vi "Login (Start Here!).vi"() -> ()   [LabVIEW 2012]
panel:
  out "error out":errorcluster
  in  "stop":bool
  out "Incorrect!":bool
  out "Verified!":bool
  in  "OK":bool
  in  "Password":string
  in  "User Name":string
  # "EXO Login"
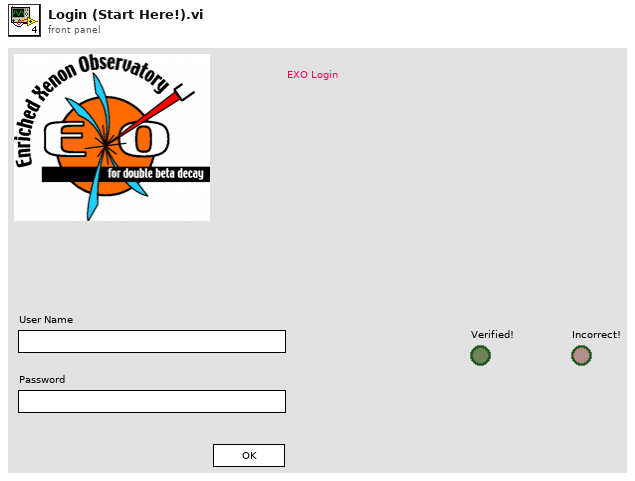
[diagram p1: front panel]
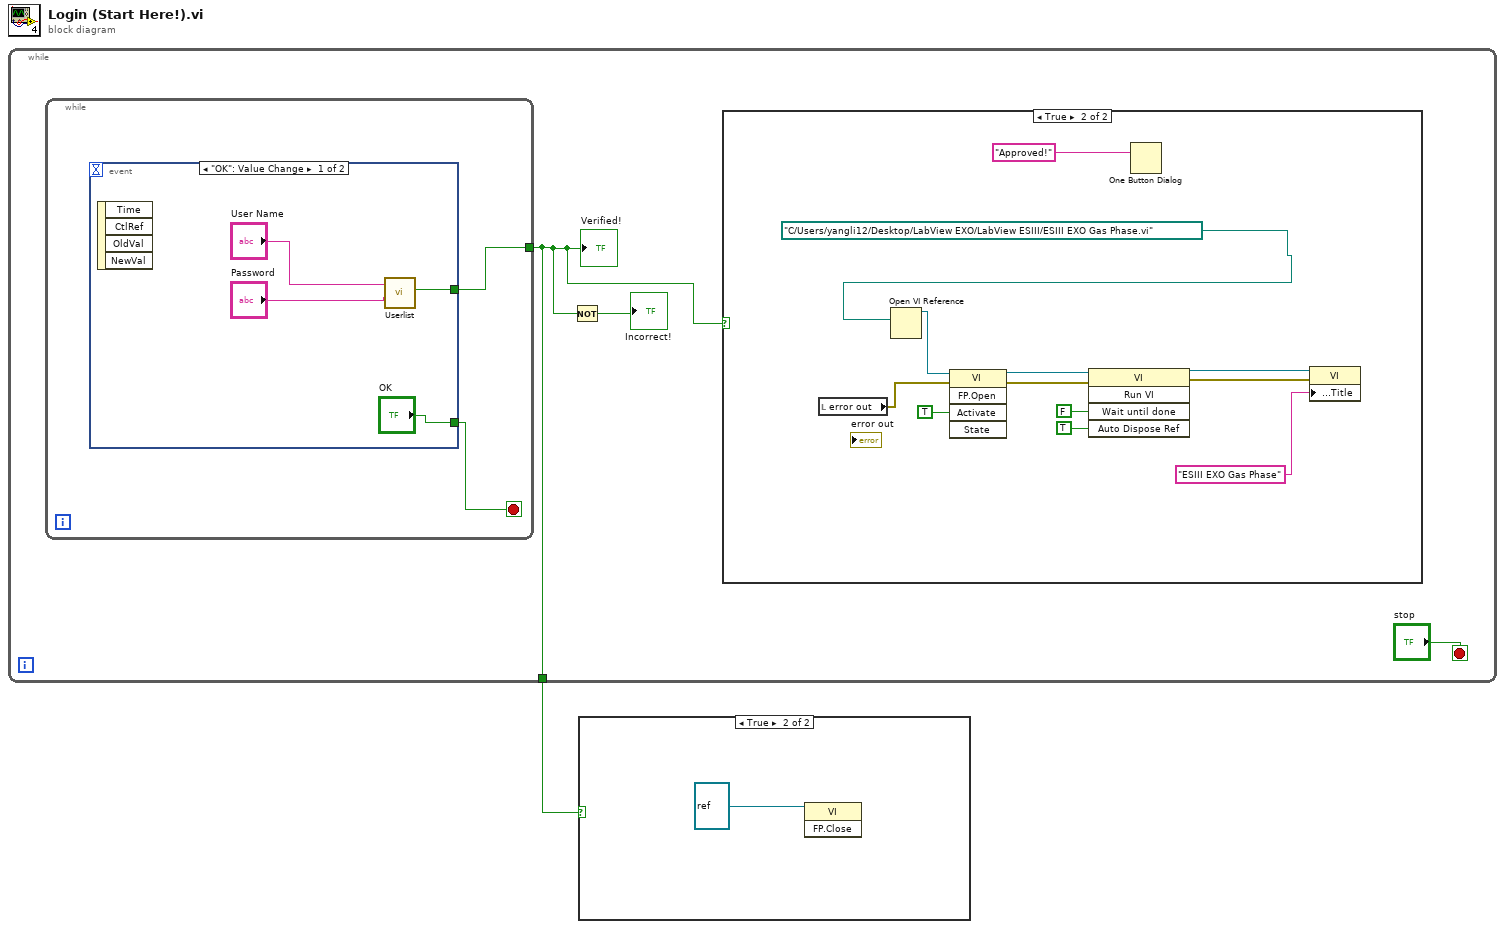
[diagram p0: block diagram]
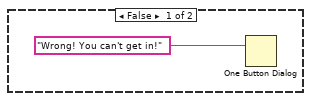
[diagram p3: hidden frame]
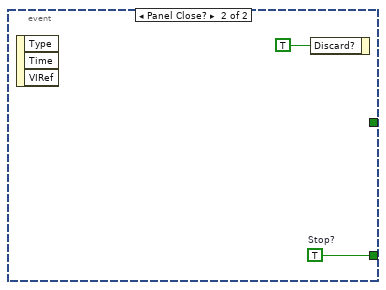
[diagram p4: hidden frame]
diagram:
  n1 = while {
    tunnel: [w2] -> w1
    stop <- "stop" stop-if-true
    n2 = while {
      tunnel: [w19] -> w2
      stop <- w18 stop-if-true
      n3 = event shown="[0] \"OK\": Value Change" {
        selector: _ -> [_ _]
        dyn-events: _ -> [_ _]
        timeout: _ -> [_ _]
        tunnel: ["OK" w24] -> w18
        tunnel: [w20 _] -> w19
        event "OK": Value Change {
          n4 = event-data() -> ()  [unwired: 1 in, 4 out]
          n5 = call "Userlist.vi"("Password"="Password", "Login"="User Name") -> ("Verified?"=w20:bool)  [unwired: 9 in]
        }
        event Panel Close? {
          w24 = TRUE  # Stop?
          n6 = event-data() -> ()  [unwired: 1 in, 3 out]
          n7 = event-data("Discard?"=TRUE) -> ()  [unwired: 1 in, 1 out]
        }
      }
    }
    "Verified!" <- w2
    n8 = Not(x=w2) -> (.not. x?=→"Incorrect!":bool)
    n9 = case shown="True" w2 {
      frame False {
        n10 = One Button Dialog(message="Wrong! You can't get in!" ("String 2")) -> ()  [unwired: 2 out]
      }
      frame True {
        n11 = local read "error out"() -> (w13:errorcluster)
        n12 = Open VI Reference(vi path=path "C:/Users/yangli12/Desktop/LabView EXO/LabView ESIII/ESIII EXO Gas Phase.vi") -> (vi reference=w16:refnum<vi>)  [unwired: 5 in, 1 out]
        n13 = invoke class="VI" method="FP.Open"(reference=w16, error in=w13, "Activate"=TRUE ("Activate?")) -> (reference out=w14:refnum<vi>, error out=w12:errorcluster)  [unwired: 2 in, 3 out]
        n14 = invoke class="VI" method="Run VI"(reference=w14, error in=w12, "Wait until done"=FALSE ("Wait Until Done"), "Auto Dispose Ref"=TRUE ("Auto Dispose Reference")) -> (reference out=w8:refnum<vi>, error out=w9:errorcluster)  [unwired: 1 in, 3 out]
        n15 = One Button Dialog(message="Approved!" ("String 2")) -> ()  [unwired: 2 out]
        n16 = property class="VI"(reference=w8, error in=w9, "Front Panel.Title"="ESIII EXO Gas Phase" ("Front Panel Window:Title")) -> ()  [unwired: 2 out]
      }
    }
  }
  n17 = case shown="True" w1 {
    frame False {
    }
    frame True {
      n18 = invoke class="VI" method="FP.Close"(reference=refnum<vi> refnum) -> ()  [unwired: 2 in, 3 out]
    }
  }
